vi "判断字符串为空.vi"(1 "字符串":string) -> (0 "为空？":bool)   [LabVIEW 2014]
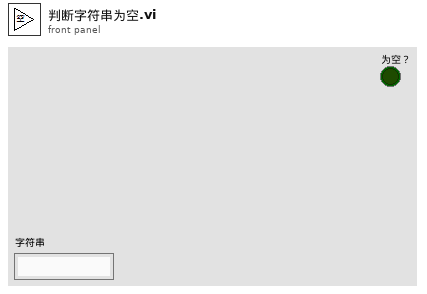
[diagram p1: front panel]
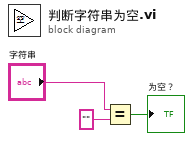
[diagram p0: block diagram]
diagram:
  n1 = Equal?(x="字符串", y="") -> (x = y?=→"为空？":bool)
